vi "Scope - size of final 5%.vi"(11 "Scope time axis":dbl[](array[numeric])) -> (1 "95% of scope time":dbl, 2 "max scope time":dbl, 3 "Size of final 5% of scope time":dbl)   [LabVIEW 2017, in "Processing.lvlib"]
uses:
  Processing.lvlib
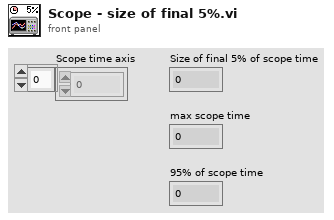
[diagram p1: front panel]
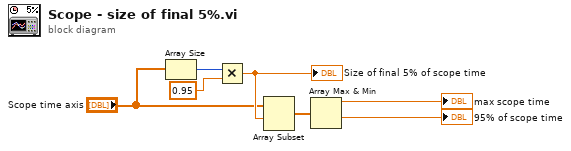
[diagram p0: block diagram]
diagram:
  n1 = Array Size(array="Scope time axis") -> (size(s)=w6:i32)
  n2 = Multiply(x=w6, y=0.95) -> (x*y=w5:dbl)
  "Size of final 5% of scope time" <- w5
  n3 = Array Subset "Array Subset"(array="Scope time axis", index=w5) -> (w4:dbl[])  [unwired: 1 in]
  n4 = Array Max & Min(array=w4) -> (max value=→"max scope time":dbl, min value=→"95% of scope time":dbl)  [unwired: 2 out]
